vi "Create Queue MWave#2.vi"(8 "error in":errorcluster) -> (0 "error out":errorcluster, 3 "queMWave#2":refnum<queue>)   [LabVIEW 2016]
uses:
  Library/Event/Ctl/EventVariantData.ctl
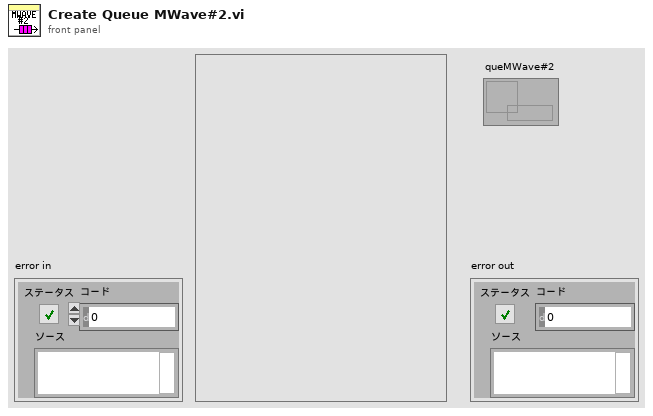
[diagram p1: front panel]
types:
  T1 = typedef "EventVariantData.ctl" = cluster{"コマンド":string, "バリアント":variant}
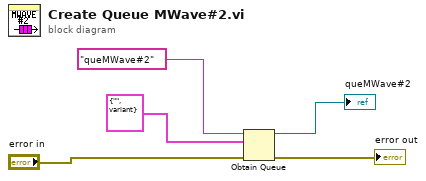
[diagram p0: block diagram]
diagram:
  n1 = Obtain Queue(name (unnamed)="queMWave#2" ("名前（名前なし）"), element data type=T1 {"コマンド"="", "バリアント"=variant}, error in (no error)="error in") -> (queue out=→"queMWave#2":refnum<queue>, error out=→"error out":errorcluster)  [unwired: 2 in, 1 out]
